vi "tmpWaves.vi"(8 "queue in":refnum<queue>, 9 "queue in":refnum<queue>, 10 "reference":refnum<vi>, 11 "Boolean in":refnum<vi>) -> (0 "Mirror Z 4":refnum<k21>, 1 "Numeric 3":i32, 2 "Mirror Z 3":refnum<k21>, 3 "Queue out":refnum<queue>, 4 "Duration":string, 5 "queue out 4":refnum<queue>, 6 "Numeric 2":i32, 7 "Mirror Z 2":refnum<k21>)   [LabVIEW 2016]
uses:
  controls/Hardware.ctl
  <vilib>/Waveform/DWDTOps.llb/DWDT Append Digital Samples.vi
  <vilib>/Waveform/WDTOps.llb/WDT Append Waveforms DBL.vi
  <vilib>/Waveform/WDTOps.llb/WDT Waveform Duration DBL.vi
  controls/ModeEnum.ctl
  controls/Microscope Settings.ctl
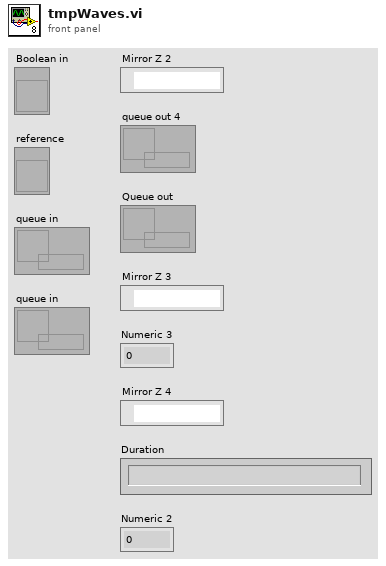
[diagram p1: front panel]
types:
  T1 = typedef "ModeEnum.ctl" = enum16{"Idle", "Init", "generateWaves", "runWaves", "runWavesCont", "endWavesCont", "stop"}
  T2 = typedef "Microscope Settings.ctl" = cluster{"Mode":enum16{"Brightfield", "X", "XY", "XYZ", "XYZT", "XYZC", "Tweezers", "Virus"}, "Slit":cluster{"Scanning Mode":dbl, "Slit Width /%":dbl}, "Colour":cluster{"Laser":enum16{"Brightfield", "445", "488", "561", "647"}, "Filter":u16}[], "Exposure/ms":dbl, "Piezo Position /um":dbl, "ROI":cluster{"X":cluster{"Start /px":dbl, "Step /px":dbl, "Range /px":dbl}, "Y":cluster{"Start /px":dbl, "Step /px":dbl, "Range /px":dbl}, "Z ":cluster{"Start /um":dbl, "Step/um":dbl, "Range /um":dbl}, "T ":cluster{"Start /s":dbl, "Step /s":dbl, "Range /s":dbl}}, "Samples per millisecond":dbl, "Relax/ms":dbl, "Readout Direction":dbl, "Trigger Source":dbl, "Camera Delay /ms":dbl, "Under Scan /ms":dbl, "Calibration Coordinates":cluster{"Top Left":dbl[], "Top Right":dbl[], "Bottom Left":dbl[], "Bottom Right":dbl[], "Waveforms":cluster{"Analogue Out":waveform(dbl)[], "Digital Out":digitalwaveform[]}}}
  T3 = typedef "Hardware.ctl" = enum16{"Stop", "RunCont", "EndCont", "Idle", "Update", "Run Waves"}
  T4 = cluster{"Laser":enum16{"Brightfield", "445", "488", "561", "647"}, "Filter":u16}[]
  T5 = enum16{"Brightfield", "X", "XY", "XYZ", "XYZT", "XYZC", "Tweezers", "Virus"}
  T6 = cluster{"Start /um":dbl, "Step/um":dbl, "Range /um":dbl}
  T7 = cluster{"Analogue Out out":waveform(dbl)[], "Digital Out out":digitalwaveform[]}
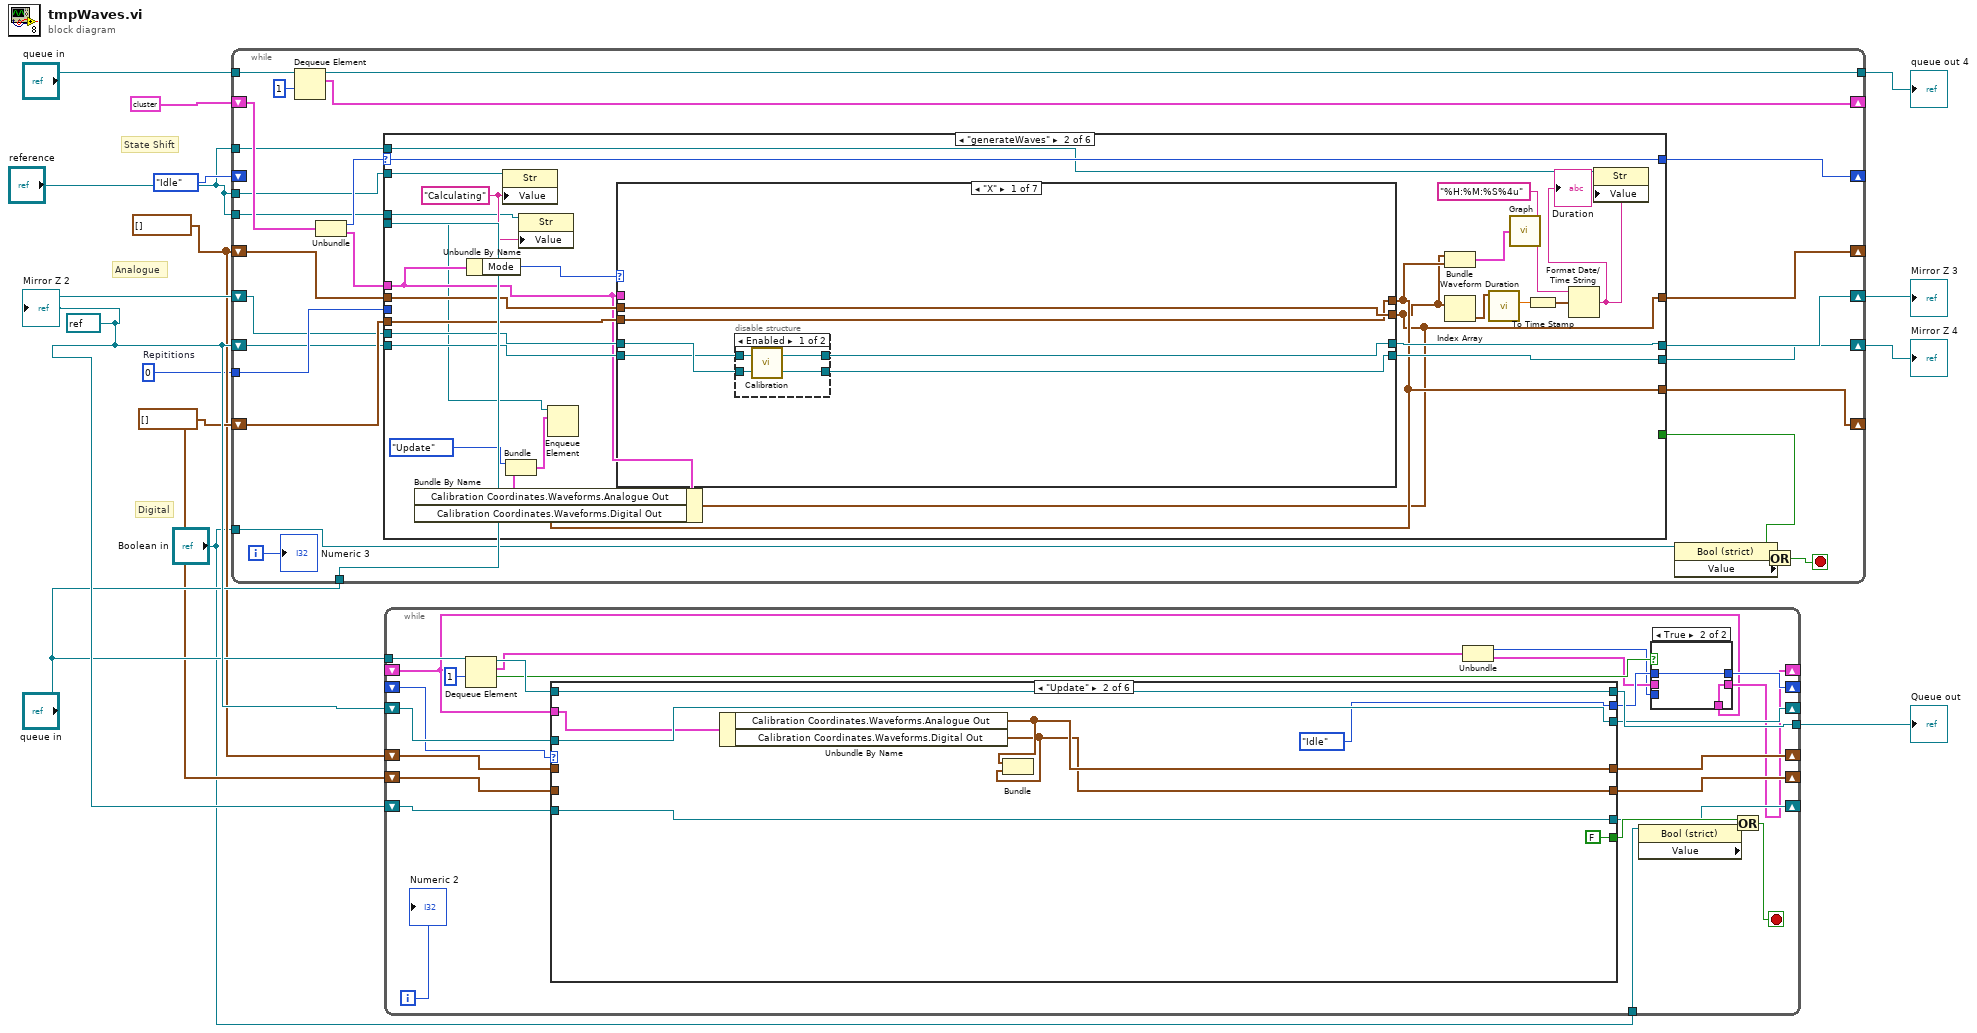
[diagram p0: block diagram]
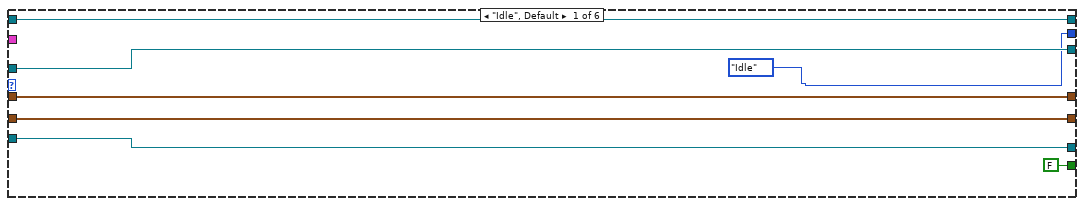
[diagram p3: hidden frame]
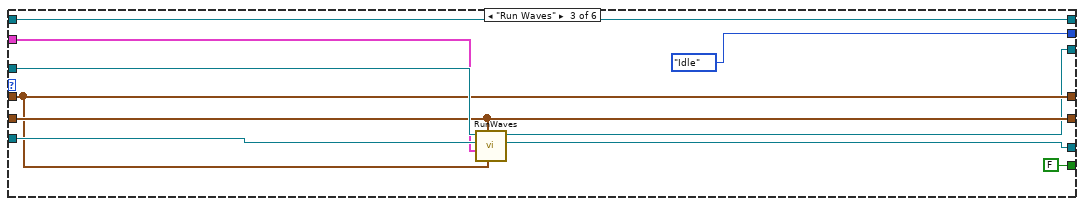
[diagram p4: hidden frame]
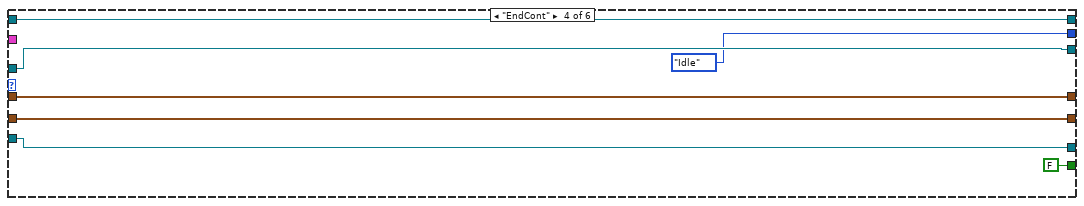
[diagram p5: hidden frame]
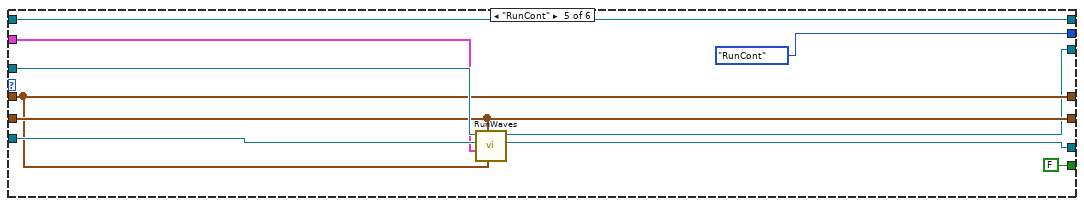
[diagram p6: hidden frame]
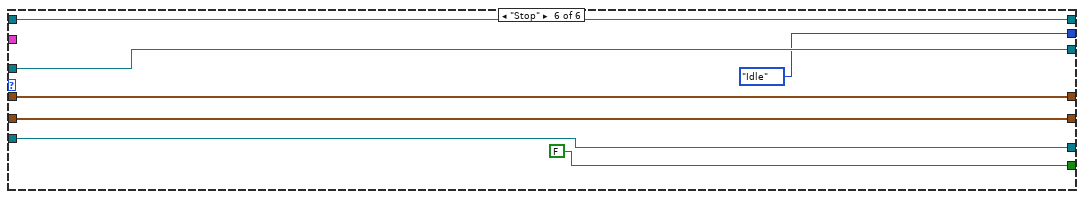
[diagram p7: hidden frame]
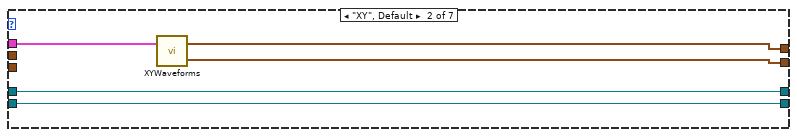
[diagram p10: hidden frame]
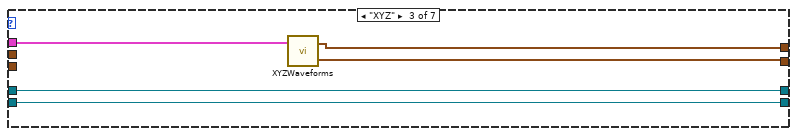
[diagram p11: hidden frame]
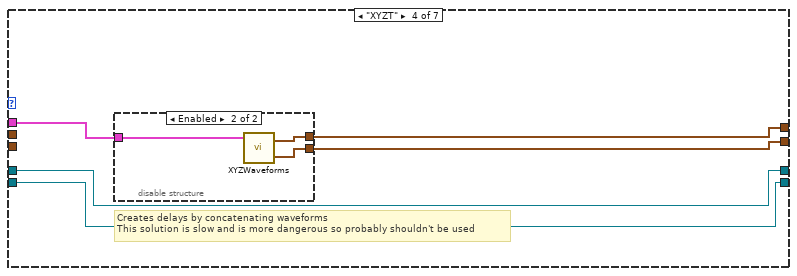
[diagram p12: hidden frame]
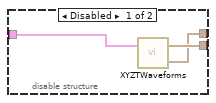
[diagram p13: hidden frame]
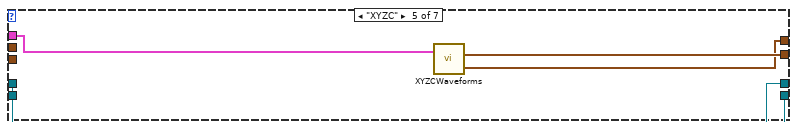
[diagram p14: hidden frame]
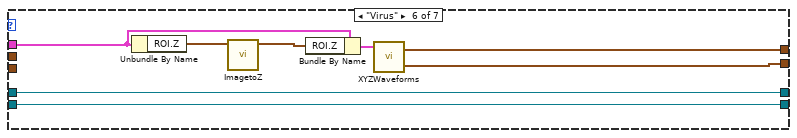
[diagram p15: hidden frame]
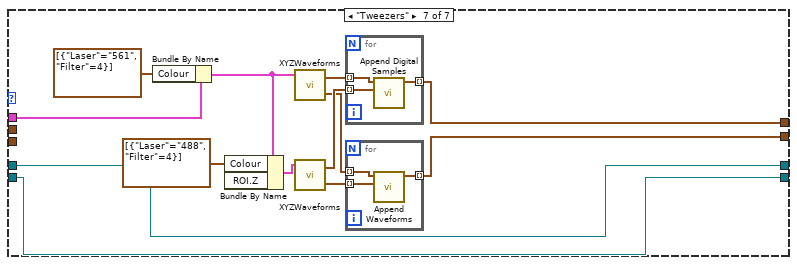
[diagram p16: hidden frame]
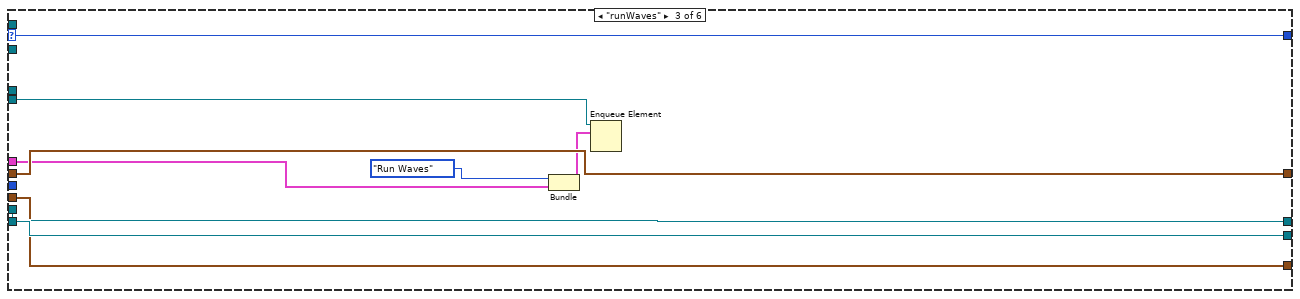
[diagram p17: hidden frame]
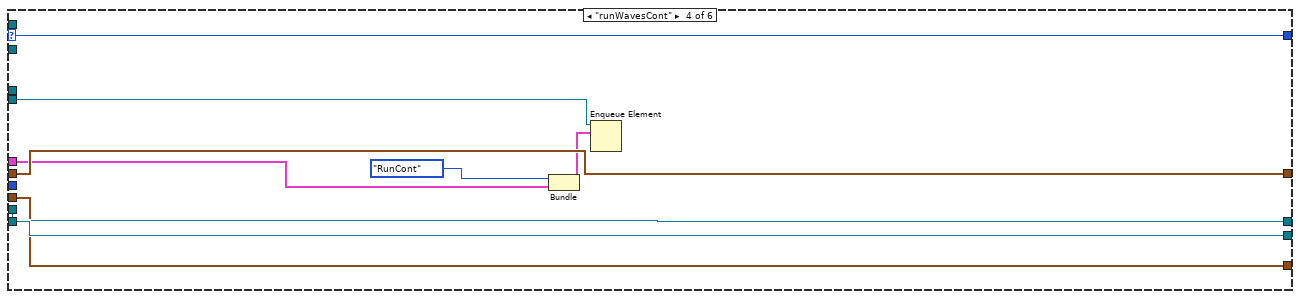
[diagram p18: hidden frame]
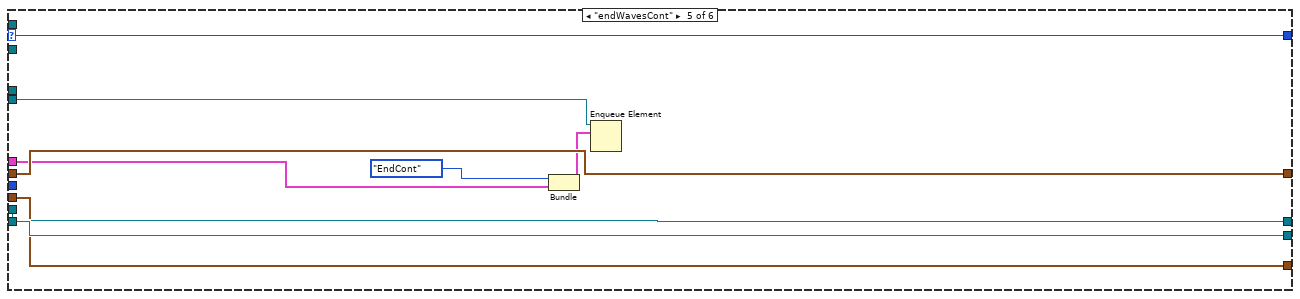
[diagram p19: hidden frame]
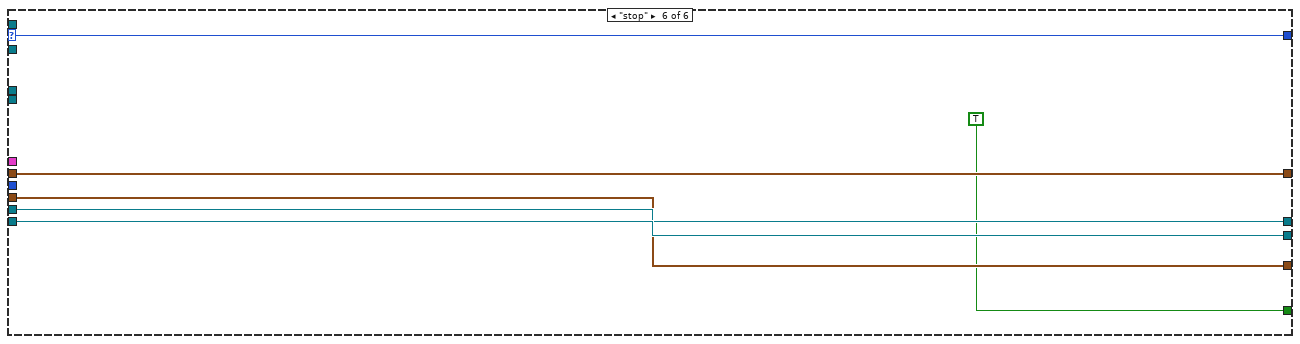
[diagram p20: hidden frame]
diagram:
  w14 = refnum<k21> refnum ("Mirror Z 2")
  w9 = digitalwaveform[] [] ("Digital Out")
  w8 = waveform(dbl)[] [] ("Analogue Out")
  w3 = 0  # Repititions
  # "State Shift"
  # "Digital"
  # "Analogue"
  n1 = while {
    tunnel: "queue in" -> [w40]
    shift-right: [w39] -> _
    shift-left: w8 -> [w38]
    tunnel: w3 -> [w37]
    shift-right: [w33] -> w5
    shift-left: w14 -> [w32]
    shift-right: [w36] -> _
    shift-left: w9 -> [w35]
    shift-right: [w31] -> w4
    shift-left: w14 -> [w30]
    tunnel: [w29] -> w6
    shift-right: [w25] -> _
    shift-left: ModeEnum."Idle" ("Mode") -> [_]
    tunnel: "queue in" -> [w22]
    shift-right: [w20] -> _
    shift-left: cluster{"Mode":T1, "Microscope Settings":T2} {"Mode"=enum."Idle", "Microscope Settings"={"Mode"=enum."X", "Slit"={"Scanning Mode"=0.0, "Slit Width /%"=0.0}, "Colour"=[], "Exposure/ms"=0.0, "Piezo Position /um"=0.0, "ROI"={"X"={"Start /px"=0.0, "Step /px"=0.0, "Range /px"=0.0}, "Y"={"Start /px"=0.0, "Step /px"=0.0, "Range /px"=0.0}, "Z "={"Start /um"=0.0, "Step/um"=0.0, "Range /um"=0.0}, "T "={"Start /s"=0.0, "Step /s"=0.0, "Range /s"=0.0}}, "Samples per millisecond"=0.0, "Relax/ms"=0.0, "Readout Direction"=0.0, "Trigger Source"=0.0, "Camera Delay /ms"=0.0, "Under Scan /ms"=0.0, "Calibration Coordinates"={"Top Left"=[], "Top Right"=[], "Bottom Left"=[], "Bottom Right"=[], "Waveforms"={"Analogue Out"=[], "Digital Out"=[]}}}} -> [w19]
    tunnel: "reference" -> [w18]
    tunnel: "reference" -> [w17]
    tunnel: "reference" -> [w16]
    tunnel: "Boolean in" -> [w15]
    i -> [w21]
    stop <- w26 stop-if-true
    n2 = Dequeue Element(queue=w40, timeout in ms (-1)=1) -> (queue out=w29:refnum<queue>, element=w20:cluster{"Mode":T1, "Microscope Settings":T2})  [unwired: 1 in, 2 out]
    n3 = Unbundle(w19) -> ("Mode"=w24:T1, "Microscope Settings"=w23:T2)
    n4 = case shown="\"generateWaves\"" w24 {
      selector: w24 -> [w41 w57 w143 w152 w161 w164]
      tunnel: [_ _ _ _ _ TRUE] -> w28
      tunnel: w23 -> [_ w56 w139 w148 w157 _]
      tunnel: [w45 w52 w141 w150 w159 w169] -> w39
      tunnel: w38 -> [w45 w68 w141 w150 w159 w169]
      tunnel: w37 -> [_ _ _ _ _ _]
      tunnel: [w42 w58 w145 w154 w163 w168] -> w31
      tunnel: [w43 w60 w144 w153 w162 w167] -> w33
      tunnel: w32 -> [w43 w61 w144 w153 w162 w167]
      tunnel: [w44 w53 w140 w149 w158 w166] -> w36
      tunnel: w35 -> [w44 w70 w140 w149 w158 w166]
      tunnel: w30 -> [w42 w59 w145 w154 w163 w168]
      tunnel: [w41 w57 w143 w152 w161 w164] -> w25
      tunnel: w22 -> [_ w54 w142 w151 w160 _]
      tunnel: w18 -> [_ w48 _ _ _ _]
      tunnel: w17 -> [_ w47 _ _ _ _]
      tunnel: w16 -> [_ w46 _ _ _ _]
      frame "Idle", Default {
      }
      frame "generateWaves" {
        w63 = "Calculating" ("date/time string")
        n5 = Unbundle By Name(w56) -> ("Mode"=w69:T5)
        n6 = property on="Property Node" class="Str"(reference=w47, "Value"=w63) -> ()  [unwired: 1 in, 2 out]
        n7 = property class="Str"(reference=w48, "Value"=w63) -> ()  [unwired: 1 in, 2 out]
        n8 = case shown="\"X\"" w69 {
          tunnel: [w76 w86 w89 w97 w108 w113 w118] -> w52
          tunnel: w56 -> [_ w87 w90 w95 w104 w112 w127]
          tunnel: [w75 w85 w88 w96 w107 w114 w121] -> w53
          tunnel: w70 -> [w75 _ _ _ _ _ _]
          tunnel: w68 -> [w76 _ _ _ _ _ _]
          tunnel: w61 -> [w74 w84 w92 w94 w106 w116 w130]
          tunnel: w59 -> [w73 w83 w91 w93 w105 w115 w129]
          tunnel: [w72 w84 w92 w94 w106 w116 w130] -> w60
          tunnel: [w71 w83 w91 w93 w105 w115 w129] -> w58
          frame "X" {
            n9 = disable-structure shown="Enabled" {
              disable-tunnel: w74 -> [w80 w81]
              disable-tunnel: w73 -> [w79 w82]
              disable-tunnel: [w78 w82] -> w72
              disable-tunnel: [w77 w81] -> w71
              frame Enabled {
                n10 = call "Calibration.vi"("Analogue In"=w80, "Digital In"=w79) -> ("Analogue In Out"=w77:refnum<k21>, "Digital Out"=w78:refnum<k21>)
              }
              frame Disabled {
              }
            }
          }
          frame "XY", Default {
            n11 = call "XYWaveforms.vi"("Microscope Settings"=w87) -> ("Analogue Out"=w86:waveform(dbl)[], "Digital Out"=w85:digitalwaveform[])  [unwired: 1 out]
          }
          frame "XYZ" {
            n12 = call "XYZWaveforms.vi"("Microscope Settings"=w90) -> ("Analogue Out out"=w89:waveform(dbl)[], "Digital Out out"=w88:digitalwaveform[])  [unwired: 2 in]
          }
          frame "XYZT" {
            # "Creates delays by concatenating waveforms\nThis solution is slow and is more dangerous so probably shouldn't be used"
            n13 = disable-structure shown="Enabled" {
              disable-tunnel: [w100 w101] -> w97
              disable-tunnel: [w99 w102] -> w96
              disable-tunnel: w95 -> [w98 w103]
              frame Disabled {
                n14 = call "XYZTWaveforms.vi"("Microscope Settings"=w98) -> ("Digital Out"=w99:digitalwaveform[], "Analogue Out"=w100:waveform(dbl)[])  [unwired: 1 in]
              }
              frame Enabled {
                n15 = call "XYZWaveforms.vi"("Microscope Settings"=w103) -> ("Analogue Out out"=w101:waveform(dbl)[], "Digital Out out"=w102:digitalwaveform[])  [unwired: 2 in]
              }
            }
          }
          frame "XYZC" {
            n16 = call "XYZCWaveforms.vi"("Microscope Settings"=w104) -> ("Array"=w107:digitalwaveform[], "Analogue Out out"=w108:waveform(dbl)[])  [unwired: 1 in]
          }
          frame "Virus" {
            n17 = Unbundle By Name(w112) -> ("ROI.Z"=w110:T6)
            n18 = call "ImagetoZ.vi"("Z"=w110) -> ("ROI.Z"=w109:T6)  [unwired: 10 in]
            n19 = Bundle By Name(cluster=w112, "ROI.Z"=w109) -> (w111:T2)
            n20 = call "XYZWaveforms.vi"("Microscope Settings"=w111) -> ("Analogue Out out"=w113:waveform(dbl)[], "Digital Out out"=w114:digitalwaveform[])  [unwired: 2 in]
          }
          frame "Tweezers" {
            n21 = Bundle By Name(cluster=w127, "Colour"=T4 [{"Laser"=enum."561", "Filter"=4}]) -> (w125:T2)
            n22 = Bundle By Name(cluster=w125, "Colour"=T4 [{"Laser"=enum."488", "Filter"=4}]) -> (w124:T2, "ROI.Z"=w117:T6)
            n23 = call "XYZWaveforms.vi"("Microscope Settings"=w125) -> ("Analogue Out out"=w120:waveform(dbl)[], "Digital Out out"=w123:digitalwaveform[])  [unwired: 2 in]
            n24 = call "XYZWaveforms.vi"("Microscope Settings"=w124) -> ("Analogue Out out"=w119:waveform(dbl)[], "Digital Out out"=w122:digitalwaveform[])  [unwired: 2 in]
            n25 = for {
              tunnel: w122 -> [w135] mode=indexing
              tunnel: w123 -> [w136] mode=indexing
              tunnel: [w134] -> w121 mode=indexing
              n26 = call-poly <vilib>:"Append Digital Samples.vi"("digital waveform B"=w135, "digital waveform A"=w136) -> ("digital waveform out"=w134:digitalwaveform)  [unwired: 8 in, 1 out]
            }
            n27 = for {
              tunnel: w119 -> [w132] mode=indexing
              tunnel: w120 -> [w133] mode=indexing
              tunnel: [w131] -> w118 mode=indexing
              n28 = call-poly <vilib>:"Append Waveforms.vi"("waveform B"=w132, "waveform A"=w133) -> ("waveform out"=w131:waveform(dbl))  [unwired: 8 in, 1 out]
            }
          }
        }
        n29 = Bundle By Name(cluster=w56, "Calibration Coordinates.Waveforms.Analogue Out"=w52, "Calibration Coordinates.Waveforms.Digital Out"=w53) -> (w55:T2)
        n30 = Bundle(Hardware."Update", "Microscope Settings"=w55) -> (w51:cluster{T3, "Microscope Settings":T2})  [unwired: 1 in]
        n31 = Enqueue Element(queue=w54, element=w51) -> ()  [unwired: 2 in, 3 out]
        n32 = Bundle("Analogue Out out"=w52, "Digital Out out"=w53) -> (w49:T7)  [unwired: 1 in]
        n33 = Index Array(array=w52) -> (element=w67:waveform(dbl))  [unwired: 1 in]
        n34 = call-poly <vilib>:"Waveform Duration.vi"("waveform in"=w67) -> ("duration"=w65:dbl)  [unwired: 8 in, 2 out]
        n35 = call "Graph.vi"("Cluster"=w49) -> ()
        n36 = To Time Stamp(1:w65) -> (0:w66:timestamp)
        n37 = Format Date/Time String(time format string (%c)="%H:%M:%S%4u", seconds (now)=w66) -> (date/time string=w62:string)  [unwired: 1 in]
        "Duration" <- w62
        n38 = property on="Property Node" class="Str"(reference=w46, "Value"=w62) -> ()  [unwired: 1 in, 2 out]
      }
      frame "runWaves" {
        n39 = Bundle(Hardware."Run Waves", "Microscope Settings"=w139) -> (w138:cluster{T3, "Microscope Settings":T2})  [unwired: 1 in]
        n40 = Enqueue Element(queue=w142, element=w138) -> ()  [unwired: 2 in, 3 out]
      }
      frame "runWavesCont" {
        n41 = Bundle(Hardware."RunCont", "Microscope Settings"=w148) -> (w147:cluster{T3, "Microscope Settings":T2})  [unwired: 1 in]
        n42 = Enqueue Element(queue=w151, element=w147) -> ()  [unwired: 2 in, 3 out]
      }
      frame "endWavesCont" {
        n43 = Bundle(Hardware."EndCont", "Microscope Settings"=w157) -> (w156:cluster{T3, "Microscope Settings":T2})  [unwired: 1 in]
        n44 = Enqueue Element(queue=w160, element=w156) -> ()  [unwired: 2 in, 3 out]
      }
      frame "stop" {
      }
    }
    n45 = property class="Bool (strict)"(reference=w15) -> ("Value"=w27:bool)  [unwired: 1 in, 2 out]
    n46 = Or(x=w28, y=w27) -> (x .or. y?=w26:bool)
    "Numeric 3" <- w21
  }
  "queue out 4" <- w6
  "Mirror Z 3" <- w5
  "Mirror Z 4" <- w4
  n47 = while {
    tunnel: [w194] -> w10
    tunnel: "queue in" -> [w193]
    shift-right: [w190] -> _
    shift-left: w8 -> [w188]
    shift-right: [w189] -> _
    shift-left: w9 -> [w187]
    shift-right: [w181] -> _
    shift-left: w14 -> [w183]
    shift-right: [w182] -> _
    shift-left: w14 -> [w184]
    shift-right: [w176] -> _
    shift-left: _ -> [w178]
    shift-right: [w173] -> _
    shift-left: _ -> [w171]
    tunnel: "Boolean in" -> [w170]
    i -> [w180]
    stop <- w186 stop-if-true
    n48 = Dequeue Element(queue=w193, timeout in ms (-1)=1) -> (queue out=w192:refnum<queue>, element=w191:cluster{T3, "Microscope Settings":T2}, timed out?=w177:bool)  [unwired: 1 in, 1 out]
    n49 = case shown="\"Update\"" w178 {
      tunnel: [w206 w214 w216 w228 w233 w246] -> w194
      tunnel: w192 -> [w206 w214 w216 w228 w233 w246]
      tunnel: w171 -> [_ w210 w220 _ w237 _]
      tunnel: [w205 w209 w221 w230 w238 w248] -> w190
      tunnel: [w204 w208 w222 w231 w239 w247] -> w189
      tunnel: w188 -> [w205 _ w221 w230 w238 w248]
      tunnel: w187 -> [w204 _ w222 w231 w239 w247]
      tunnel: [FALSE FALSE FALSE FALSE FALSE FALSE] -> w185
      tunnel: w184 -> [w203 w213 w224 w227 w241 w244]
      tunnel: w183 -> [w202 w212 w223 w226 w240 w243]
      tunnel: [w203 w213 w219 w227 w236 w244] -> w182
      tunnel: [w202 w212 w218 w226 w235 w243] -> w181
      tunnel: [Hardware."Idle" Hardware."Idle" Hardware."Idle" Hardware."Idle" Hardware."RunCont" Hardware."Idle"] -> w175
      frame "Idle", Default {
      }
      frame "Update" {
        n50 = Unbundle By Name(w210) -> ("Calibration Coordinates.Waveforms.Analogue Out"=w209:waveform(dbl)[], "Calibration Coordinates.Waveforms.Digital Out"=w208:digitalwaveform[])
        n51 = Bundle("Analogue Out"=w209, "Digital Out"=w208) -> ()  [unwired: 1 in, 1 out]
      }
      frame "Run Waves" {
        n52 = call "RunWaves.vi"("Analogue Out"=w221, "Digital Out"=w222, "Microscope Settings"=w220, "Mirror Z in"=w223, "Refnum in"=w224) -> ("task out"=w218:refnum<k21>, "Refnum out"=w219:refnum<k21>)  [unwired: 5 in]
      }
      frame "EndCont" {
      }
      frame "RunCont" {
        n53 = call "RunWaves.vi"("Analogue Out"=w238, "Digital Out"=w239, "Microscope Settings"=w237, "Mirror Z in"=w240, "Refnum in"=w241) -> ("task out"=w235:refnum<k21>, "Refnum out"=w236:refnum<k21>)  [unwired: 5 in]
      }
      frame "Stop" {
      }
    }
    n54 = Unbundle(w191) -> (w172:T3, "Microscope Settings"=w174:T2)
    n55 = property class="Bool (strict)"(reference=w170) -> ("Value"=w195:bool)  [unwired: 1 in, 2 out]
    n56 = case shown="True" w177 {
      tunnel: [w196 w199] -> w176
      tunnel: w175 -> [_ w199]
      tunnel: [w197 w198] -> w173
      tunnel: w174 -> [w197 _]
      tunnel: w172 -> [w196 _]
      tunnel: w171 -> [_ w198]
      frame False {
      }
      frame True {
      }
    }
    n57 = Or(x=w185, y=w195) -> (x .or. y?=w186:bool)
    "Numeric 2" <- w180
  }
  "Queue out" <- w10
  "Mirror Z 2" <- w14
